vi "measVoltCompleteTrig.vi"() -> (1 "Connector1/DIO31":bool, 2 "Connector1/DIO30":bool, 3 "PXI_Trigger_4_out":bool)   [LabVIEW 2014]
uses:
  measVoltGlobVars.vi
  <vilib>/rvi/eio/common/nirviEmuTemplateMethod_errors.vi
  <vilib>/eio/EIONode/EIONode.xnode
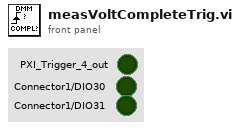
[diagram p1: front panel]
types:
  T1 = typedef "measVoltCompleteDest.ctl" = enum16{"PT4", "C1D30", "C1D31", "PT4_C1D30", "PT4_C1D31", "PT4_C1D30_C1D31", "C1D30_C1D31", "software"}
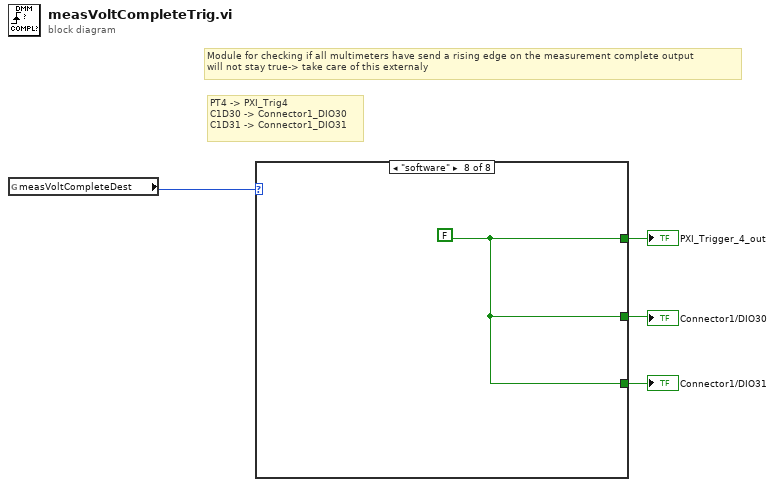
[diagram p0: block diagram]
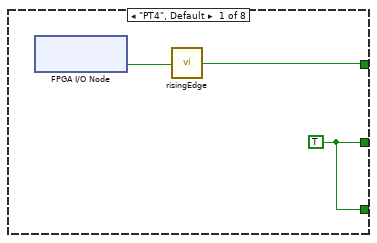
[diagram p2: hidden frame]
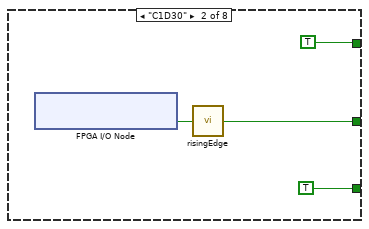
[diagram p3: hidden frame]
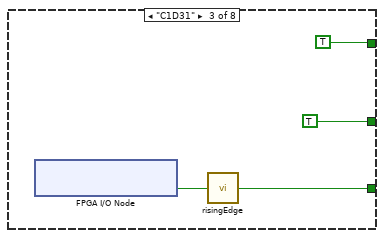
[diagram p4: hidden frame]
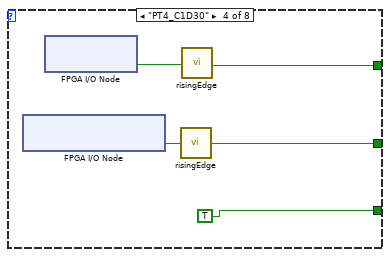
[diagram p5: hidden frame]
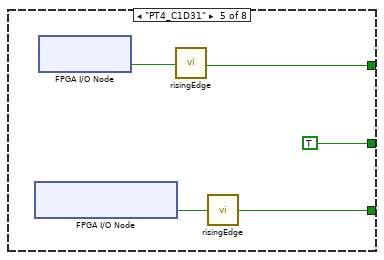
[diagram p6: hidden frame]
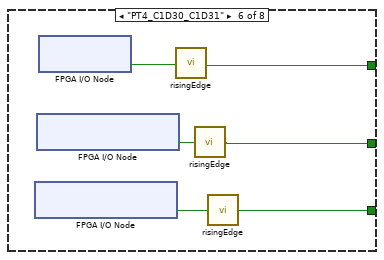
[diagram p7: hidden frame]
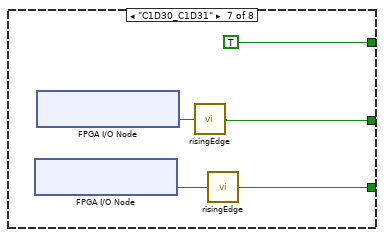
[diagram p8: hidden frame]
diagram:
  # "Module for checking if all multimeters have send a rising edge on the measurement complete output\nwill not stay true-> take care of this externaly"
  # "PT4 -> PXI_Trig4\nC1D30 -> Connector1_DIO30\nC1D31 -> Connector1_DIO31"
  n1 = global read "measVoltGlobVars.vi" "measVoltCompleteDest"() -> (w4:T1)
  n2 = case shown="\"software\"" w4 {
    tunnel: [w6 TRUE TRUE w19 w21 w28 TRUE ("out") w37] -> w3
    tunnel: [w5 w8 TRUE w16 TRUE w26 w33 w37] -> w2
    tunnel: [w5 TRUE w13 TRUE w24 w30 w35 w37] -> w1
    frame "PT4", Default {
      w5 = TRUE
      n3 = xnode "FPGA I/O Node"() -> ("PXI_Trig4"=w7:bool)  [unwired: 1 in, 1 out]
      n4 = call "risingEdge.vi"("In"=w7) -> ("out"=w6:bool)
    }
    frame "C1D30" {
      n5 = xnode "FPGA I/O Node"() -> ("Connector1/DIO30"=w11:bool)  [unwired: 1 in, 1 out]
      n6 = call "risingEdge.vi"("In"=w11) -> ("out"=w8:bool)
    }
    frame "C1D31" {
      n7 = xnode "FPGA I/O Node"() -> ("Connector1/DIO31"=w14:bool)  [unwired: 1 in, 1 out]
      n8 = call "risingEdge.vi"("In"=w14) -> ("out"=w13:bool)
    }
    frame "PT4_C1D30" {
      n9 = xnode "FPGA I/O Node"() -> ("Connector1/DIO30"=w17:bool)  [unwired: 1 in, 1 out]
      n10 = xnode "FPGA I/O Node"() -> ("PXI_Trig4"=w20:bool)  [unwired: 1 in, 1 out]
      n11 = call "risingEdge.vi"("In"=w17) -> ("out"=w16:bool)
      n12 = call "risingEdge.vi"("In"=w20) -> ("out"=w19:bool)
    }
    frame "PT4_C1D31" {
      n13 = xnode "FPGA I/O Node"() -> ("Connector1/DIO31"=w25:bool)  [unwired: 1 in, 1 out]
      n14 = xnode "FPGA I/O Node"() -> ("PXI_Trig4"=w22:bool)  [unwired: 1 in, 1 out]
      n15 = call "risingEdge.vi"("In"=w22) -> ("out"=w21:bool)
      n16 = call "risingEdge.vi"("In"=w25) -> ("out"=w24:bool)
    }
    frame "PT4_C1D30_C1D31" {
      n17 = xnode "FPGA I/O Node"() -> ("Connector1/DIO31"=w31:bool)  [unwired: 1 in, 1 out]
      n18 = xnode "FPGA I/O Node"() -> ("Connector1/DIO30"=w27:bool)  [unwired: 1 in, 1 out]
      n19 = xnode "FPGA I/O Node"() -> ("PXI_Trig4"=w29:bool)  [unwired: 1 in, 1 out]
      n20 = call "risingEdge.vi"("In"=w29) -> ("out"=w28:bool)
      n21 = call "risingEdge.vi"("In"=w27) -> ("out"=w26:bool)
      n22 = call "risingEdge.vi"("In"=w31) -> ("out"=w30:bool)
    }
    frame "C1D30_C1D31" {
      n23 = xnode "FPGA I/O Node"() -> ("Connector1/DIO31"=w36:bool)  [unwired: 1 in, 1 out]
      n24 = xnode "FPGA I/O Node"() -> ("Connector1/DIO30"=w34:bool)  [unwired: 1 in, 1 out]
      n25 = call "risingEdge.vi"("In"=w34) -> ("out"=w33:bool)
      n26 = call "risingEdge.vi"("In"=w36) -> ("out"=w35:bool)
    }
    frame "software" {
      w37 = FALSE
    }
  }
  "PXI_Trigger_4_out" <- w3
  "Connector1/DIO30" <- w2
  "Connector1/DIO31" <- w1
